vi "SL TAGS Single Tag to Value.vi"(4 "Tag":T1) -> (1 "Tag Value":T9)   [LabVIEW 2017, in "EEISysLink.lvclass"]
doc: "Input a class tag and convert to a class tag value.\n\nJames Tillett P.E.\nEndeavor Engineering Inc.\nwww.endeavoreng.com"
uses:
  EEISysLink.lvclass
  Controls/SL Tag Value.ctl
  Controls/SL Tag Data Type.ctl
  Controls/SL Tag.ctl
  <vilib>/Skyline/Tag/Wrapper/Wrapper_class/NI Skyline Tag.lvclass
  Controls/SL Tag Properties.ctl
  Controls/SL Tag Interpolation Method.ctl
  Controls/SL Tag Unit of Measure.ctl
  Controls/SL Tag Type.ctl
  <vilib>/Skyline/Tag/Shared/typedefs/Tag Cluster.ctl
  <vilib>/Skyline/Tag/Shared/typedefs/DataType.ctl
  <vilib>/Skyline/Tag/Shared/NI Skyline Tag.lvlib
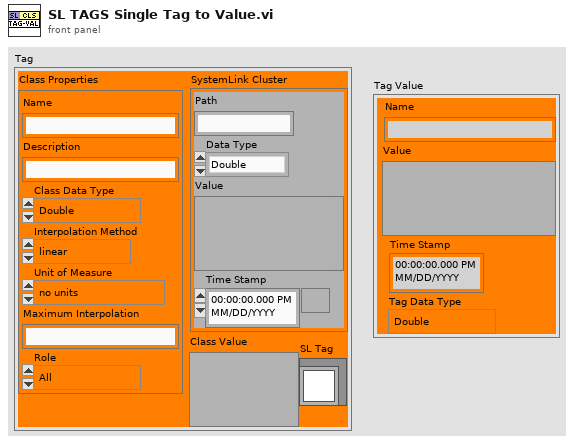
[diagram p1: front panel]
types:
  T1 = typedef "EEISysLink.lvclass/SL Tag.ctl" = cluster{"Class Properties":T2, "SL Tag":refnum<class "NI Skyline Tag.lvclass">, "SystemLink Cluster":T7, "Class Value":variant}
  T2 = typedef "EEISysLink.lvclass/SL Tag Properties.ctl" = cluster{"Class Data Type":T3, "Name":string, "Description":string, "Interpolation Method":T4, "Unit of Measure":T5, "Maximum Interpolation":string, "Role":T6}
  T3 = typedef "EEISysLink.lvclass/SL Tag Data Type.ctl" = enum16{"Double", "Integer", "String", "Boolean", "Waveform"}
  T4 = typedef "EEISysLink.lvclass/SL Tag Interpolation Method.ctl" = enum16{"linear", "pilinear", "step"}
  T5 = typedef "EEISysLink.lvclass/SL Tag Unit of Measure.ctl" = enum16{"no units", "Second", "Hour", "Minute", "Day", "Year", "Month", "Week", "Foot", "Yard", "Meter", "Centimeter", "Inch", "Mile", "Nautical Mile", "Miles per Hour", "Meters per second", "Square meter", "Cubic meter", "Cubic centimeter", "Cubic inch", "Liter", "Gallon", "Gallons dry US", "Gallon UK", "Percent", "Revolutions per minute", "Revolution", "Degree angle", "Astronomical Unit", "Atom", "Atomic mass", "Bar", "Byte", "C (speed of light)", "Curie", "Decibel", "Electron Volt", "Ounce", "Knot", "G", "Grade", "Are", "Hectare", "Faraday", "Franklin", "Gilbert", "Erg", "Lambert", "Maxwell", "Gauss", "Electron mass", "Kilogram force", "Pound force", "Rad", "Centiradian", "Sphere", "Mach", "Fluid Ounces", "Fluid Ounces UK", "Fahrenheit", "Celsius", "Kelvin", "Rankine", "Gram", "Kilogram", "Pound", "Short/US Ton", "Long/UK ton", "Metric ton", "Mole", "Pounds per square inch", "Inches water column", "Torr", "Millitorr", "Millimeter mercury", "Inches mercury", "Bar (2)", "Atmosphere", "Pascal", "Watt", "kiloWatt", "Horsepower", "Kilowatt Hour", "British thermal units", "Millions of BTU", "Ampere", "Candela", "Radian", "Steradian", "Bit", "Hertz", "Newton", "Joule", "Coulomb", "Volt", "Farad", "Ohm", "Siemens", "Weber", "Tesla", "Henry", "Lumen", "Lux", "Becqueral", "Gray", "Sievert", "Katal", "Angstrom", "Light Year", "Parsec", "Point", "Pixel", "Dyne", "Kilogram force (2)", "Pound force (2)", "Rem", "Rutherford", "Roentgen"}
  T6 = typedef "EEISysLink.lvclass/SL Tag Type.ctl" = enum16{"All", "Supervisor", "Worker"}
  T7 = typedef "NI Skyline Tag.lvlib/Tag Cluster.ctl" = cluster{"Path":string, "Data Type":T8, "Value":variant, "Time Stamp":timestamp}
  T8 = typedef "NI Skyline Tag.lvlib/DataType.ctl" = enum32{"Double", "Integer", "String"}
  T9 = typedef "SL Tag Value.ctl" = cluster{"Value":variant, "Time Stamp":timestamp, "Tag Data Type":T3, "Name":string}
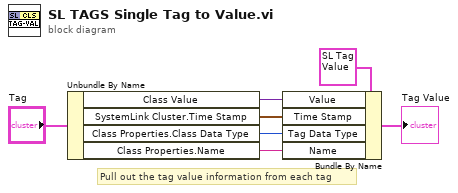
[diagram p0: block diagram]
diagram:
  # "Pull out the tag value information from each tag"
  n1 = Unbundle By Name("Tag") -> ("Class Value"=w2:variant, "SystemLink Cluster.Time Stamp"=w3:timestamp, "Class Properties.Class Data Type"=w4:T3, "Class Properties.Name"=w5:string)
  n2 = Bundle By Name(cluster=T9 {"Value"=variant, "Time Stamp"=timestamp(0 s since 1904-01-01), "Tag Data Type"=enum."Double", "Name"=""} ("Tag Value"), "Value"=w2, "Time Stamp"=w3, "Tag Data Type"=w4, "Name"=w5) -> (→"Tag Value":T9)
